vi "digital read all.vi"(8 "error in (no error)":errorcluster, 11 "USB-6000 in":refnum<class "USB-6000.lvclass">) -> (0 "error out":errorcluster, 2 "data":bool[](array[boolean]), 3 "USB-6000 out":refnum<class "USB-6000.lvclass">)   [LabVIEW 2025, in "USB IO.lvlib" / "USB-6000.lvclass"]
uses:
  USB-6000.lvclass
  USB-6000.lvclass/USB-6000.ctl
  <vilib>/DAQmx/read.llb/DAQmx Read (Digital 1D Bool 1Chan 1Samp).vi
  <vilib>/DAQmx/miscellaneous.llb/DAQmx Fill In Error Info.vi
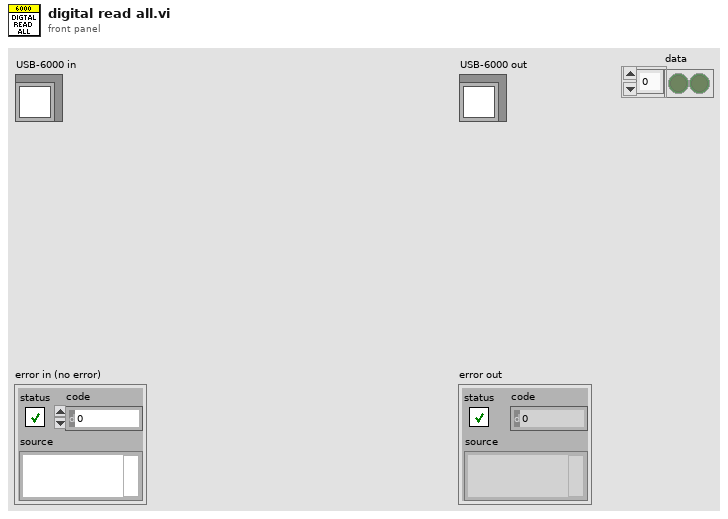
[diagram p1: front panel]
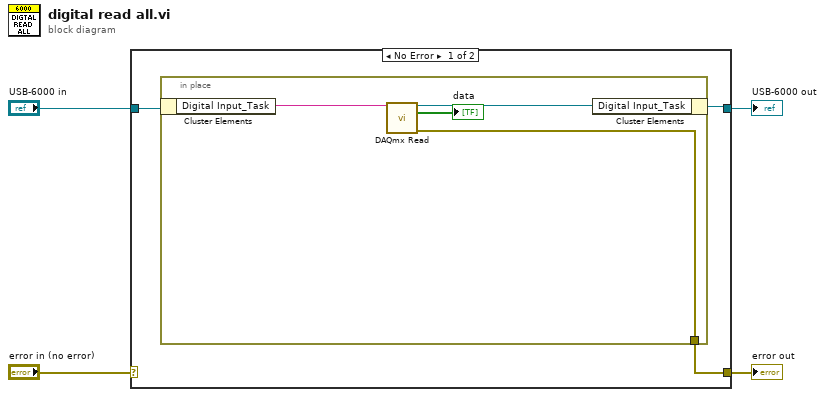
[diagram p0: block diagram]
diagram:
  n1 = case shown="No Error" "error in (no error)" {
    selector: "error in (no error)" -> [_ w13]
    tunnel: [w5 w13] -> w3
    tunnel: [w6 w12] -> w1
    tunnel: "USB-6000 in" -> [w7 w12]
    frame No Error {
      n2 = in-place {
        in-place-border: [w9] -> w5
        n3 = in-place-cluster #1(w7) -> ("Digital Input_Task"=w11:string)
        n4 = call-poly <vilib>:"DAQmx Read.vi"("task/channels in"=w11) -> ("task out"=w10:refnum<k21>, "data"=→"data":bool[], "error out"=w9:errorcluster)  [unwired: 12 in]
        n5 = in-place-cluster #1("Digital Input_Task"=w10) -> (w6:refnum<class "USB-6000.lvclass">)
      }
    }
    frame Error {
    }
  }
  "error out" <- w3
  "USB-6000 out" <- w1
